vi "new.vi"() -> ()   [LabVIEW 2019]
uses:
  <vilib>/myRIO/Common/Instrument Driver Framework/myRIO v1.0/Encoder/typedefs/Encoder Signal Mode.ctl
  <vilib>/myRIO/Instrument Drivers/Onboard IO/Encoder/typedefs/Encoder Reference.ctl
  <vilib>/myRIO/Common/Instrument Driver Framework/Utilities/typedefs/myRIO Generic Hardware Reference.ctl
  <vilib>/myRIO/Common/Instrument Driver Framework/Utilities/typedefs/Hardware Version Enum.ctl
  <vilib>/myRIO/Common/Instrument Driver Framework/Utilities/typedefs/myRIO v1.0 Reference.ctl
  <vilib>/myRIO/Common/Instrument Driver Framework/Utilities/typedefs/Generic FPGA Reference.ctl
  <vilib>/myRIO/Common/Instrument Driver Framework/myRIO v1.0/Encoder/typedefs/Encoder Channels Enum.ctl
  <vilib>/myRIO/Common/Instrument Driver Framework/myRIO v1.0/Encoder/typedefs/Encoder Configuration v1.0.ctl
  <vilib>/userDefined/High Color/nirio_resource_hc.ctl
  <vilib>/myRIO/Common/Instrument Driver Framework/Utilities/vis/Is FPGA Ref Available.vi
  <vilib>/myRIO/Common/Instrument Driver Framework/myRIO v1.0/Encoder/vis/myRIO v1.1 Open Encoder.vi
  <vilib>/myRIO/Instrument Drivers/Onboard IO/Encoder/vis/Read.vi
  <vilib>/myRIO/Common/Instrument Driver Framework/Utilities/vis/Validate Channels.vi
  <vilib>/myRIO/Common/Instrument Driver Framework/myRIO v1.0/Encoder/vis/myRIO v1.0 Reserve Encoder.vi
  <vilib>/myRIO/Common/Instrument Driver Framework/myRIO v1.0/UART/vis/myRIO v1.0 Close UART.vi
  <vilib>/myRIO/Common/Instrument Driver Framework/myRIO v1.0/Encoder/vis/myRIO v1.0 Build MUX Configuration Encoder.vi
  <vilib>/myRIO/Common/Instrument Driver Framework/myRIO v1.0/Resource Manager/vis/myRIO v1.0 Reserve Channel List.vi
  <vilib>/myRIO/Common/Instrument Driver Framework/myRIO v1.0/Resource Manager/vis/myRIO v1.0 Create Configuration List.vi
  <vilib>/myRIO/Common/Instrument Driver Framework/myRIO v1.0/Resource Manager/vis/myRIO v1.0 Reserve Channel.vi
  <vilib>/myRIO/Common/Instrument Driver Framework/myRIO v1.0/Resource Manager/vis/myRIO v1.0 Unreserve Channel.vi
  <vilib>/myRIO/Common/Instrument Driver Framework/myRIO v1.0/Resource Manager/vis/myRIO v1.0 Build Mutex Name.vi
  <vilib>/Utility/VariantDataType/GetNumericInfo.vi
  <vilib>/Utility/error.llb/Error Cluster From Error Code.vi
  <vilib>/myRIO/Common/Instrument Driver Framework/myRIO v1.0/myRIO v1.1 Open.vi
  <vilib>/myRIO/Common/Instrument Driver Framework/Utilities/vis/IO Manager.vi
  <vilib>/myRIO/Common/Instrument Driver Framework/Utilities/vis/Configuration Manager.vi
  <vilib>/myRIO/Common/Instrument Driver Framework/myRIO v1.0/Resource Manager/vis/myRIO v1.0 Configure IO.vi
  <vilib>/myRIO/Common/Instrument Driver Framework/myRIO v1.0/myRIO v1.0 Close.vi
  <vilib>/myRIO/Common/Instrument Driver Framework/myRIO v1.0/Encoder/vis/myRIO v1.0 Configure Encoder.vi
  <vilib>/myRIO/Common/Instrument Driver Framework/myRIO v1.0/Encoder/vis/myRIO v1.0 Read Encoder.vi
  <vilib>/Utility/file.llb/Write Delimited Spreadsheet (DBL).vi
  <vilib>/myRIO/Common/Instrument Driver Framework/Utilities/vis/FPGA Ref Manager.vi
  <vilib>/myRIO/Common/Instrument Driver Framework/myRIO v1.0/myRIO v1.0 Reset FPGA.vi
  <vilib>/myRIO/Common/Instrument Driver Framework/myRIO v1.0/IRQ/vis/myRIO v1.0 IRQ Info FGV.vi
  <vilib>/myRIO/Common/Instrument Driver Framework/myRIO v1.0/IRQ/vis/myRIO v1.0 Timer IRQ Info FGV.vi
  <vilib>/myRIO/Common/Instrument Driver Framework/myRIO v1.0/IRQ/vis/myRIO v1.0 ISR Agent.vi
  <vilib>/myRIO/Instrument Drivers/Utilities/vis/Reset Index.vi
  <vilib>/myRIO/Common/Instrument Driver Framework/myRIO v1.0/Resource Manager/vis/myRIO v1.0 Block Write Resource Manager.vi
  <vilib>/myRIO/Express VI/Onboard IO/Encoder/Encoder Express VI.xnode
  <vilib>/myRIO/Common/Instrument Driver Framework/myRIO v1.0/Encoder/typedefs/Encoder Count Direction Enum.ctl
  <vilib>/myRIO/Instrument Drivers/Onboard IO/Encoder/vis/myRIO Encoder Open.xnode
  <vilib>/myRIO/Instrument Drivers/Onboard IO/Encoder/Encoder.lvlib
  <vilib>/myRIO/Instrument Drivers/Utilities/Utilities.lvlib
panel:
  out "error out 3":errorcluster
  in  "Stop 3":bool
  out "Direction 3":enum16{"Counting Up", "Counting Down"}(ring)
  out "Overflow? 3":bool
  in  "Reset 3":bool
  out "actual pos":dbl
  out "Graph 3":cluster{dbl, dbl}(graph)
  in  "Freq[Hz] 2":dbl=1000.0
  out "Duty Cycle":dbl=0.5
  in  "k_":dbl
  in  "b_":dbl=1.0
  in  "reference":dbl
  out "K1_c":dbl
  out "K2_c":dbl
  out "Graph 2":dbl(graph)
  out "target pos":dbl
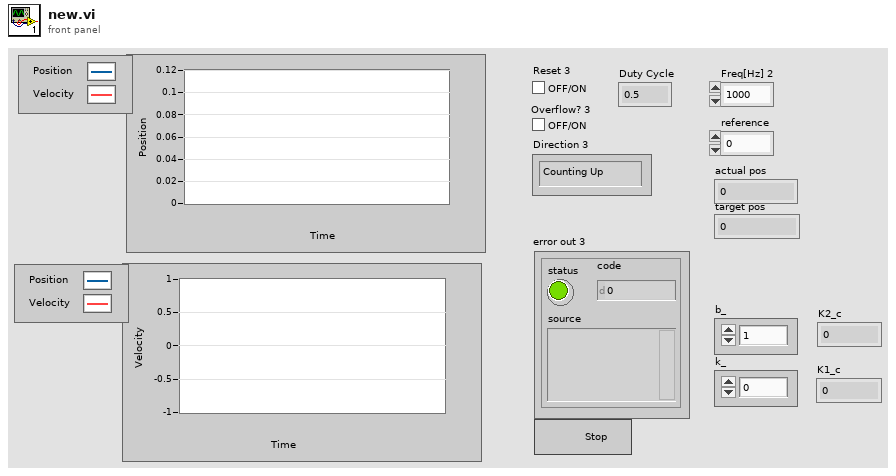
[diagram p1: front panel]
types:
  T1 = typedef "Encoder.lvlib/Encoder Reference.ctl" = cluster{"myRIO Reference":T2, "Encoder Channels Enum":T6}
  T2 = typedef "myRIO Generic Hardware Reference.ctl" = cluster{"myRIO Model":T3, "myRIO Hardware Reference":T4}
  T3 = typedef "Hardware Version Enum.ctl" = enum16{"Unknown", "myRIO-1900", "myRIO-1950", "roboRIO", "NI ELVIS RIO CM", "ELVIS III"}
  T4 = typedef "myRIO v1.0 Reference.ctl" = cluster{"Generic FPGA Reference":T5, "Allow multiple opens":bool}
  T5 = typedef "Generic FPGA Reference.ctl" = refnum<k20>
  T6 = typedef "Encoder Channels Enum.ctl" = enum16{"Not Connected", "C/ENC0", "C/ENC1", "A/ENC", "A/ENC0", "A/ENC1", "A/ENC2", "A/ENC3", "A/ENC4", "A/ENC5", "A/ENC6", "A/ENC7", "A/ENC8", "A/ENC9", "B/ENC", "B/ENC0", "B/ENC1", "B/ENC2", "B/ENC3", "B/ENC4", "B/ENC5", "B/ENC6", "B/ENC7", "B/ENC8", "B/ENC9", "DIO/ENC0", "DIO/ENC1", "DIO/ENC2", "DIO/ENC3", "DIO/ENC4"}
  T7 = typedef "Encoder Signal Mode.ctl" = enum16{"Quadrature phase signal", "Step and direction signal"}
  T8 = typedef "nirio_resource_hc.ctl" = tag
  T9 = typedef "Encoder Count Direction Enum.ctl" = enum16{"Counting Up", "Counting Down"}
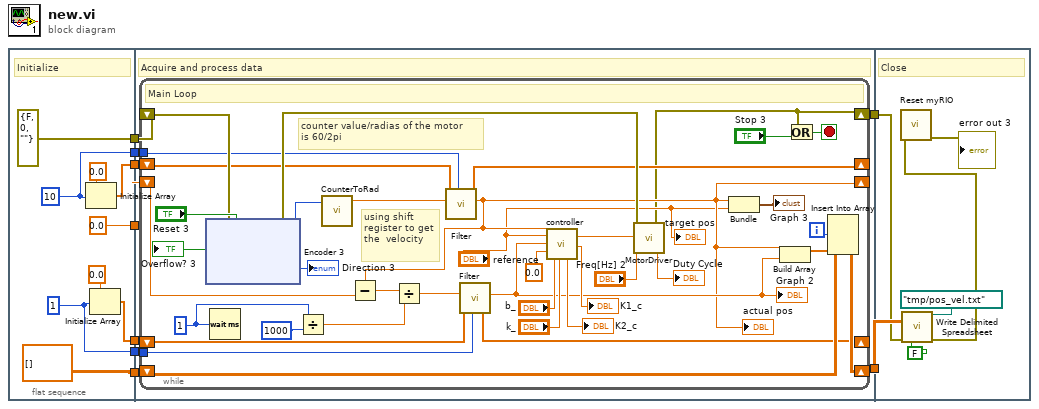
[diagram p0: block diagram]
diagram:
  n1 = flat-sequence {
    tunnel: [errorcluster {"status"=FALSE, "code"=0, "source"=""} ("error in (no error)")] -> w9
    tunnel: [0.0] -> w8
    tunnel: [dbl[][] [] ("array")] -> w7
    tunnel: [w14] -> w6
    tunnel: [w13] -> w5
    tunnel: [w11] -> w4
    tunnel: [w10] -> w3
    tunnel: w9 -> [w27]
    tunnel: w8 -> [w26]
    tunnel: w7 -> [w25]
    tunnel: [w24] -> w2
    tunnel: w6 -> [w23]
    tunnel: w5 -> [w22]
    tunnel: w4 -> [w21]
    tunnel: w3 -> [w20]
    tunnel: [w19] -> w1
    tunnel: w2 -> [w115]
    tunnel: w1 -> [w116]
    frame #0 {
      w10 = 1 ("dimension size")
      w14 = 10 ("dimension size")
      # "Initialize"
      n2 = Initialize Array(0.0 ("element"), w14) -> (w13:dbl[])
      n3 = Initialize Array(0.0 ("element"), w10) -> (w11:dbl[])
    }
    frame #1 {
      # "Acquire and process data"
      n4 = while {
        shift-right: [w28] -> w24
        shift-left: w27 -> [w49]
        shift-right: [w30] -> _
        shift-left: w26 -> [w48]
        shift-right: [w56] -> w19
        shift-left: w25 -> [w55]
        tunnel: w23 -> [w40]
        shift-right: [w38] -> _
        shift-left: w22 -> [w41]
        shift-right: [w33] -> _
        shift-left: w21 -> [w35]
        tunnel: w20 -> [w34]
        i -> [w39]
        stop <- w64 stop-if-true
        w60 = u32 1 ("milliseconds to wait")
        # "using shift register to get the  velocity"
        # "counter value/radias of the motor \nis 60/2pi"
        # "Main Loop"
        n5 = xnode "Encoder 3"("error in (no error)"=w49, "Reset Counter"="Reset 3") -> ("error out"=w51:errorcluster, "Counter Value"=w57:i32, "Counter Direction"=→"Direction 3":T9, "Overflow?"=→"Overflow? 3":bool)
        n6 = Wait (ms)(milliseconds to wait=w60) -> ()  [unwired: 1 out]
        n7 = Divide(x=w60, y=u32 1000) -> (x/y=w50:dbl)
        n8 = call "CounterToRad.vi"("Counter Value"=w57) -> ("rads"=w37:dbl)  [unwired: 10 in]
        n9 = call "Filter.vi"("data"=w37, "Buffer Len"=w40, "Buffer in"=w41) -> ("ave out"=w30:dbl, "Buffer out"=w38:dbl[])  [unwired: 7 in]
        "actual pos" <- w30
        n10 = Subtract(x=w30, y=w48) -> (x-y=w58:dbl)
        n11 = Divide(x=w58, y=w50) -> (x/y=w36:dbl)
        n12 = call "Filter.vi"("data"=w36, "Buffer Len"=w34, "Buffer in"=w35) -> ("ave out"=w31:dbl, "Buffer out"=w33:dbl[])  [unwired: 7 in]
        "Graph 2" <- w31
        n13 = call "controller.vi"("position"=w30, "pos ref"="reference", "velocity"=w31, "vel ref"=0.0, "b_"="b_", "k_"="k_") -> ("duty out"=w47:dbl, "K1_c"=→"K1_c":dbl, "K2_c"=→"K2_c":dbl)  [unwired: 11 in]
        n14 = call "MotorDriver.vi"("Frequency [Hz]"="Freq[Hz] 2", "Duty Cycle in"=w47, "error in (no error)"=w51) -> ("Duty Cycle out"=→"Duty Cycle":dbl, "error out"=w28:errorcluster)  [unwired: 10 in, 1 out]
        n15 = Bundle("ave out"=w30, "reference"="reference") -> (→"Graph 3":cluster{"ave out":dbl, "reference":dbl})  [unwired: 1 in]
        n16 = Build Array(w30, w31) -> (w54:dbl[])
        n17 = Or(x=w28, y="Stop 3") -> (x .or. y?=w64:bool)
        n18 = Insert Into Array(array=w55, index (row)=w39, new element=w54) -> (w56:dbl[][])  [unwired: 1 in]
        "target pos" <- "reference"
      }
    }
    frame #2 {
      # "Close"
      n19 = call-poly <vilib>:"Write Delimited Spreadsheet.vi"("file path (dialog if empty)"=path "/tmp/pos_vel.txt", "2D data"=w116, "error in (no error)"=w115, "transpose? (no:F)"=FALSE) -> ("error out"=w114:errorcluster)  [unwired: 10 in, 1 out]
      n20 = call <vilib>:"Reset myRIO.vi"("error in (no error)"=w114) -> ("error out"=→"error out 3":errorcluster)  [unwired: 10 in]
    }
  }
